vi "Measure_OutPut.vi"(8 "error in (no error)":errorcluster, 10 "Ring":u16(ring) items=["Voltage", "Current", "Power"], 11 "Instrument In":refnum<visa-resource-name>) -> (0 "error out":errorcluster, 2 "Measurement":dbl format="%.4g", 3 "Instrument Out":refnum<visa-resource-name>)   [LabVIEW 2022 SP3]
uses:
  <instrlib>/BK Precision 9200 Series/BK Precision 9200 Series.lvlib
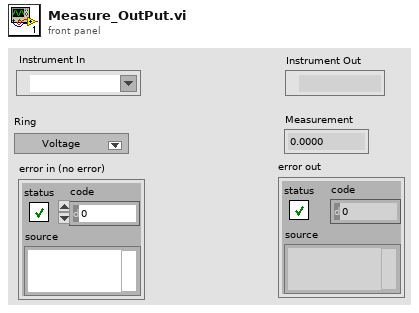
[diagram p1: front panel]
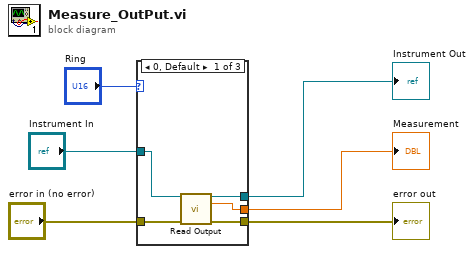
[diagram p0: block diagram]
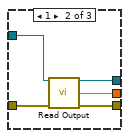
[diagram p2: hidden frame]
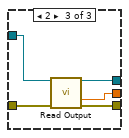
[diagram p3: hidden frame]
diagram:
  n1 = case shown="0, Default" "Ring" {
    tunnel: [w11 w16 w21] -> w6
    tunnel: "error in (no error)" -> [w10 w14 w17]
    tunnel: [w7 w15 w20] -> w1
    tunnel: "Instrument In" -> [w9 w13 w18]
    tunnel: [w8 w12 w19] -> w2
    frame 0, Default {
      n2 = call <instrlib>:"Read Output.vi"("VISA resource name"=w9, "error in (no error)"=w10) -> ("VISA resource name out"=w8:refnum<visa-resource-name>, "Actual Voltage Level (V)"=w7:dbl, "error out"=w11:errorcluster)  [unwired: 9 in, 2 out]
    }
    frame 1 {
      n3 = call <instrlib>:"Read Output.vi"("VISA resource name"=w13, "error in (no error)"=w14) -> ("VISA resource name out"=w12:refnum<visa-resource-name>, "Actual Current Level (A)"=w15:dbl, "error out"=w16:errorcluster)  [unwired: 9 in, 2 out]
    }
    frame 2 {
      n4 = call <instrlib>:"Read Output.vi"("VISA resource name"=w18, "error in (no error)"=w17) -> ("VISA resource name out"=w19:refnum<visa-resource-name>, "Actual Power Level (W)"=w20:dbl, "error out"=w21:errorcluster)  [unwired: 9 in, 2 out]
    }
  }
  "Instrument Out" <- w2
  "error out" <- w6
  "Measurement" <- w1
